vi "Sidestep Globals.vi"() -> ()   [LabVIEW 2012]
panel:
  in  "Trans Dur":dbl=1000.0
  in  "Spin Dur":dbl=1000.0
  in  "Pause Dur":dbl=250.0
  in  "X Speed":dbl=0.5
  in  "Y Speed":dbl=0.35
  in  "Back Dur":dbl=1000.0
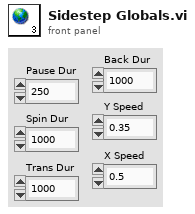
[diagram p1: front panel]
diagram:
